vi "Vehicle Position Simulation View.vi"(8 "error in (no error)":errorcluster, 11 "View Model":T1) -> (0 "error out":errorcluster)   [LabVIEW 2017]
doc: "This View used to simulate the travel of the car through the enclosure by activating Station sensors.\n[Covers: UI4]"
uses:
  Model/Controls/View Model.ctl
  Model/Controls/Shared Model.ctl
  Error Handler/Controls/Error Model.ctl
  Error Handler/Controls/Error Message.ctl
  Error Handler/Controls/Error Type.ctl
  Configuration/Controls/Config Model.ctl
  Configuration/Controls/Config DB Message.ctl
  Configuration/Controls/Config DB Command.ctl
  Configuration/Controls/Config DB Overhead.ctl
  Configuration/Controls/Config DB Record.ctl
  Controller/Controls/Controller Model.ctl
  Controls/Vehicle - Position.ctl
  Controller/Controls/Controller Overhead.ctl
  Controller/Controls/Controller Wash Step.ctl
panel:
  in  "Position":u8(slide) caption="Vehicle Position Simulation" max=4 step=1 scale=0.0..4.0
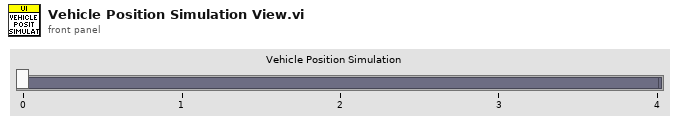
[diagram p1: front panel]
types:
  T1 = typedef "View Model.ctl" = cluster{"Shared Model":T2, "Error Model":T3, "Config Model":T4, "Controller Model":T5}
  T2 = typedef "Shared Model.ctl" = cluster{"Stop":refnum<user-event>, "Stop DVR":refnum<data-value>}
  T3 = typedef "Error Model.ctl" = cluster{"Error":refnum<user-event>}
  T4 = typedef "Config Model.ctl" = cluster{"Config":refnum<user-event>, "Config DVR":refnum<data-value>}
  T5 = typedef "Controller Model.ctl" = cluster{"Position Change":refnum<user-event>, "Overhead DVR":refnum<data-value>, "Start Wash":refnum<user-event>}
  T6 = typedef "Error Type.ctl" = enum16{"Minor Error", "Wash Cycle Error", "System Error", "Unknown"}
  T7 = typedef "Vehicle - Position.ctl" = enum16{"Entry", "Station 1", "Station 2", "Station 3", "Exit"}
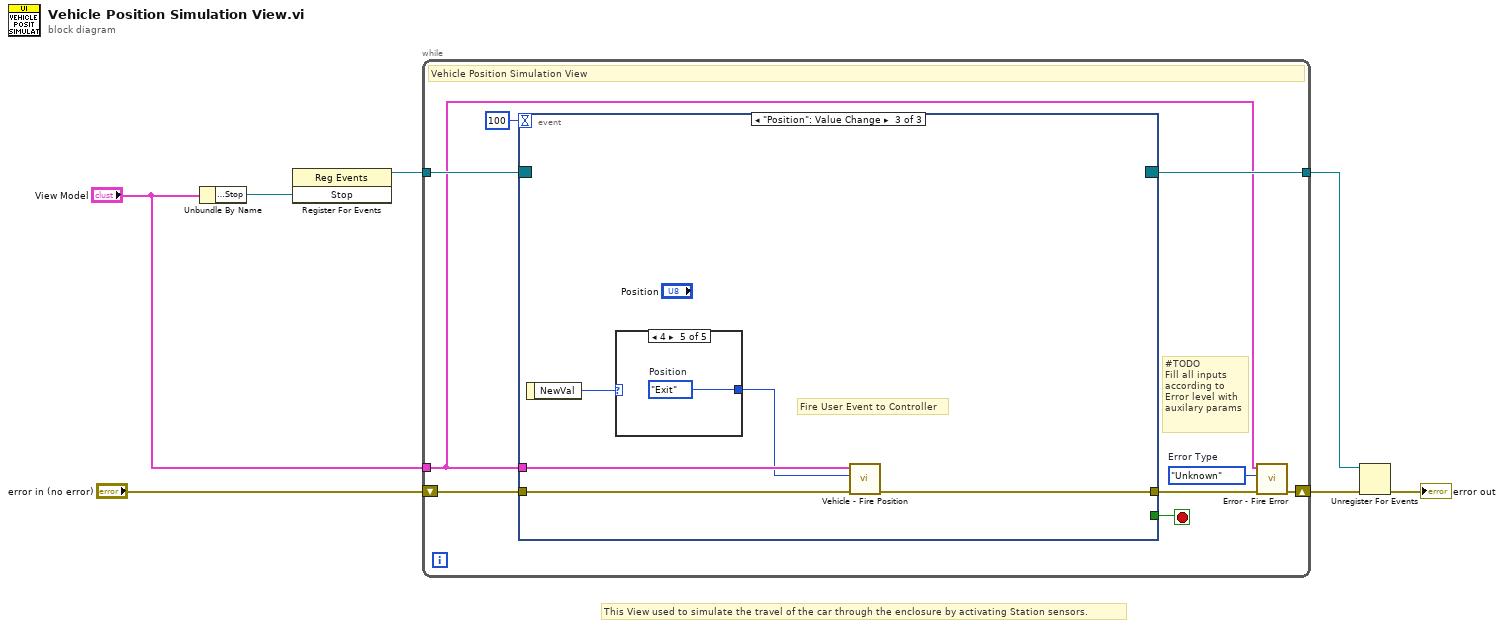
[diagram p0: block diagram]
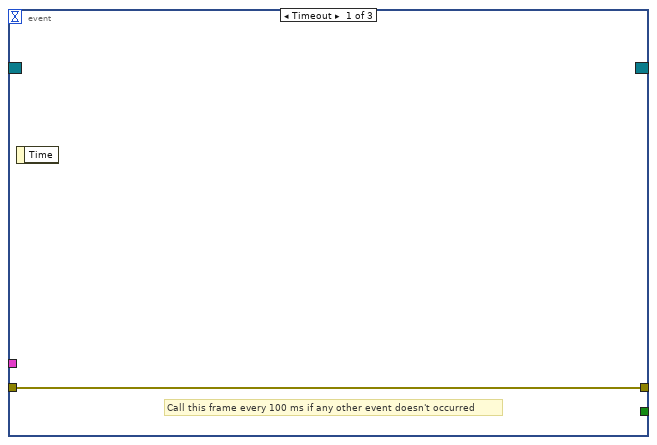
[diagram p2: hidden frame]
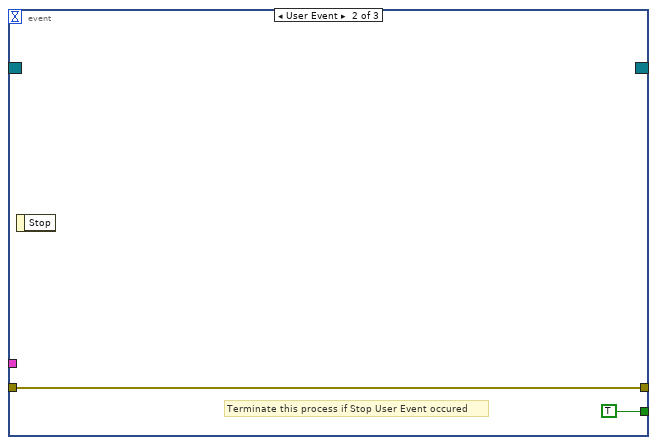
[diagram p3: hidden frame]
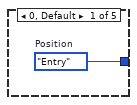
[diagram p4: hidden frame]
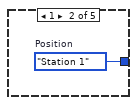
[diagram p5: hidden frame]
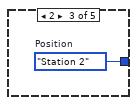
[diagram p6: hidden frame]
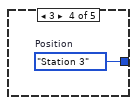
[diagram p7: hidden frame]
diagram:
  # "This View used to simulate the travel of the car through the enclosure by activating Station sensors."
  n1 = Unbundle By Name("View Model") -> ("Shared Model.Stop"=w7:refnum<user-event>)
  n2 = register-events(w7) -> (reference out=w6:refnum<event-registration>)  [unwired: 2 in, 1 out]
  n3 = while {
    tunnel: w6 -> [w16]
    shift-right: [w10] -> w4
    shift-left: "error in (no error)" -> [w14]
    tunnel: [w13] -> w2
    tunnel: "View Model" -> [w8]
    stop <- w12 stop-if-true
    w9 = Error_Type."Unknown"  # Error Type
    # "#TODO\nFill all inputs\naccording to \nError level with\nauxilary params"
    # "Vehicle Position Simulation View"
    n4 = event shown="[2] \"Position\": Value Change" {
      selector: w16 -> [_ _ _]
      dyn-events: [_ _ _] -> w13
      timeout: 100 -> [_ _ _]
      tunnel: w14 -> [w17 w19 w23]
      tunnel: [w17 w19 w22] -> w11
      tunnel: w8 -> [_ _ w21]
      tunnel: [_ TRUE _] -> w12
      event Timeout {
        # "Call this frame every 100 ms if any other event doesn't occurred"
        n5 = event-data() -> ()  [unwired: 1 in, 1 out]
      }
      event User Event {
        # "Terminate this process if Stop User Event occured"
        n6 = event-data() -> ()  [unwired: 1 in, 1 out]
      }
      event "Position": Value Change {
        # "Fire User Event to Controller"
        n7 = event-data() -> ("NewVal"=w24:u8)  [unwired: 1 in]
        n8 = case shown="4" w24 {
          tunnel: [w25 w26 w27 w28 w29] -> w20
          frame 0, Default {
            w25 = Vehicle_-_Position."Entry"  # Position
          }
          frame 1 {
            w26 = Vehicle_-_Position."Station 1"  # Position
          }
          frame 2 {
            w27 = Vehicle_-_Position."Station 2"  # Position
          }
          frame 3 {
            w28 = Vehicle_-_Position."Station 3"  # Position
          }
          frame 4 {
            w29 = Vehicle_-_Position."Exit"  # Position
          }
        }
        n9 = call "Vehicle - Fire Position.vi"("error in (no error)"=w23, "Position"=w20, "View Model"=w21) -> ("error out"=w22:errorcluster)  [unwired: 7 in, 1 out]
      }
    }
    n10 = call "Error - Fire Error.vi"("error in (no error)"=w11, "Error Type"=w9, "View Model"=w8) -> ("error out"=w10:errorcluster)  [unwired: 7 in, 1 out]
  }
  n11 = Unregister For Events(event registration refnum=w2, error in=w4) -> (error out=→"error out":errorcluster)
